vi "InitMainSize.vi"(1 "VI Refnum In":refnum<vi>) -> (0 "VI Refnum Out":refnum<vi>)   [LabVIEW 2010]
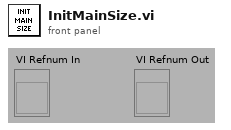
[diagram p1: front panel]
types:
  T1 = typedef "LVAllMonitorsDisplayTypeDef.ctl" = cluster{"Bounds":cluster{"Left":i16, "Top":i16, "Right":i16, "Bottom":i16}, "Depth":i16}[]
  T2 = cluster{"Bounds":cluster{"Left":i16, "Top":i16, "Right":i16, "Bottom":i16}, "Depth":i16}
  T3 = cluster{"Left":i16, "Top":i16, "Right":i16, "Bottom":i16}
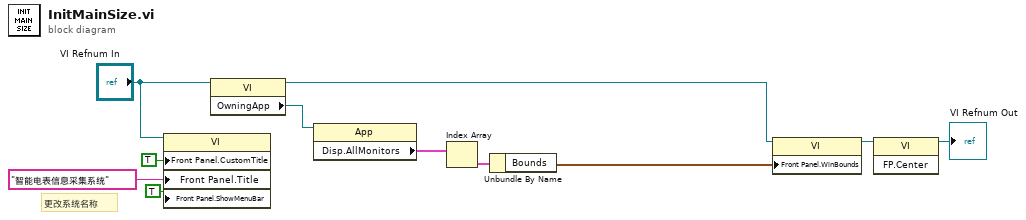
[diagram p0: block diagram]
diagram:
  # "更改系统名称"
  n1 = property class="VI"(reference="VI Refnum In", "Front Panel.CustomTitle"=TRUE ("Front Panel Window:Custom Title"), "Front Panel.Title"="智能电表信息采集系统" ("Front Panel Window:Title"), "Front Panel.ShowMenuBar"=TRUE ("Front Panel Window:Show Menu Bar")) -> ()  [unwired: 1 in, 2 out]
  n2 = property class="VI"(reference="VI Refnum In") -> (reference out=w1:refnum<vi>, "OwningApp"=w11:refnum<vi>)  [unwired: 1 in, 1 out]
  n3 = property class="App"(reference=w11) -> ("Disp.AllMonitors"=w4:T1)  [unwired: 1 in, 2 out]
  n4 = Index Array(array=w4) -> (element=w3:T2)  [unwired: 1 in]
  n5 = Unbundle By Name(w3) -> ("Bounds"=w2:T3)
  n6 = property class="VI"(reference=w1, "Front Panel.WinBounds"=w2) -> (reference out=w6:refnum<vi>)  [unwired: 1 in, 1 out]
  n7 = invoke class="VI" method="FP.Center"(reference=w6) -> (reference out=→"VI Refnum Out":refnum<vi>)  [unwired: 2 in, 2 out]
